vi "Actor Core.vi"(8 "Error In":errorcluster, 11 "BNT_SLTagMonitor in":refnum<class "BNT_SLTagMonitor.lvclass">) -> (0 "Error Out":errorcluster, 3 "Actor out":refnum<class "Actor.lvclass">)   [LabVIEW 2019, in "BNT_SLTagMonitor.lvlib" / "BNT_SLTagMonitor.lvclass"]
doc: "(<B>Filename</B>: Actor Framework.lvlib:Actor.lvclass:Actor Core.vi)\n\nReceives messages to the actor, reacts to them, and initiates any error handling that may shut the actor down.\n\nDescendant classes may override this VI to append parallel tasks for the actor to complete while it handles messages. Overrides use the Call Parent Method node."
uses:
  BNT_SLTagMonitor.lvclass
  CSPP_Core/Messages/CSPP_PVUpdate Msg/CSPP_PVUpdate Msg.lvclass
  CSPP_Core/Classes/CSPP_ProcessVariables/ProcessVariable/PV.lvclass
  CSPP_Core/Actors/CSPP_PVMonitor/CSPP_PVMonitor.lvclass
  CSPP_Core/Actors/CSPP_BaseActor/CSPP_BaseActor.lvclass
  C:/Users/Holger/Documents/LVP/CSPP/CSPP-Template/Packages/CSPP_Core/Actors/CSPP_PVMonitor/CSPP_PVMonitor.lvclass
  C:/Users/Holger/Documents/LVP/CSPP/CSPP-Template/Packages/CSPP_Core/Actors/CSPP_BaseActor/CSPP_BaseActor.lvclass
  C:/Program Files (x86)/National Instruments/LabVIEW 2019/vi.lib/ActorFramework/Actor/Actor.lvclass
  CSPP_Core/Actors/CSPP_BaseActor Messages/Open Actor Core FP Msg/Open Actor Core FP Msg.lvclass
  <vilib>/ActorFramework/Actor/Actor.lvclass
  <vilib>/Skyline/Tag/Wrapper/Wrapper_class/NI Skyline Tag.lvclass
  CSPP_Core/Libraries/Utilities/CSPP_Utilities.lvlib
  <vilib>/Skyline/Tag/Wrapper/Wrapper_class/Read Tag (Timestamp).vi
  <vilib>/Skyline/Tag/Wrapper/Wrapper_class/Read Tag (String).vi
  <vilib>/Skyline/Tag/Wrapper/Wrapper_class/Read Tag (I32).vi
  <vilib>/Skyline/Tag/Wrapper/Wrapper_class/Read Tag (DBL).vi
  <vilib>/Skyline/Tag/Wrapper/Wrapper_class/Read Tag (Boolean).vi
panel:
  out "Monitor Name":string
  out "Monitored PVs":string[](array[string])
  in  "Refresh Button":bool
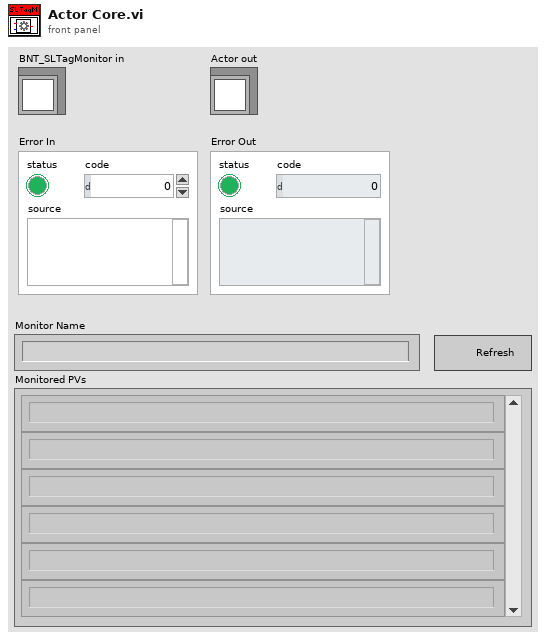
[diagram p1: front panel]
types:
  T1 = cluster{"Stop":refnum<user-event>, "PV Connections":refnum<user-event>}
  T2 = cluster{"Enqueuer":refnum<class "Message Enqueuer.lvclass">, "CSPP_PVUpdate Msg":refnum<class "CSPP_PVUpdate Msg.lvclass">}[]
  T3 = typedef "NI Skyline Tag.lvlib/DataType.ctl" = enum32{"Double", "I32", "String", "Boolean", "U64", "Timestamp"}
  T4 = cluster{"PV URL":string, "Observers":cluster{"Enqueuer":refnum<class "Message Enqueuer.lvclass">, "CSPP_PVUpdate Msg":refnum<class "CSPP_PVUpdate Msg.lvclass">}[]}[]
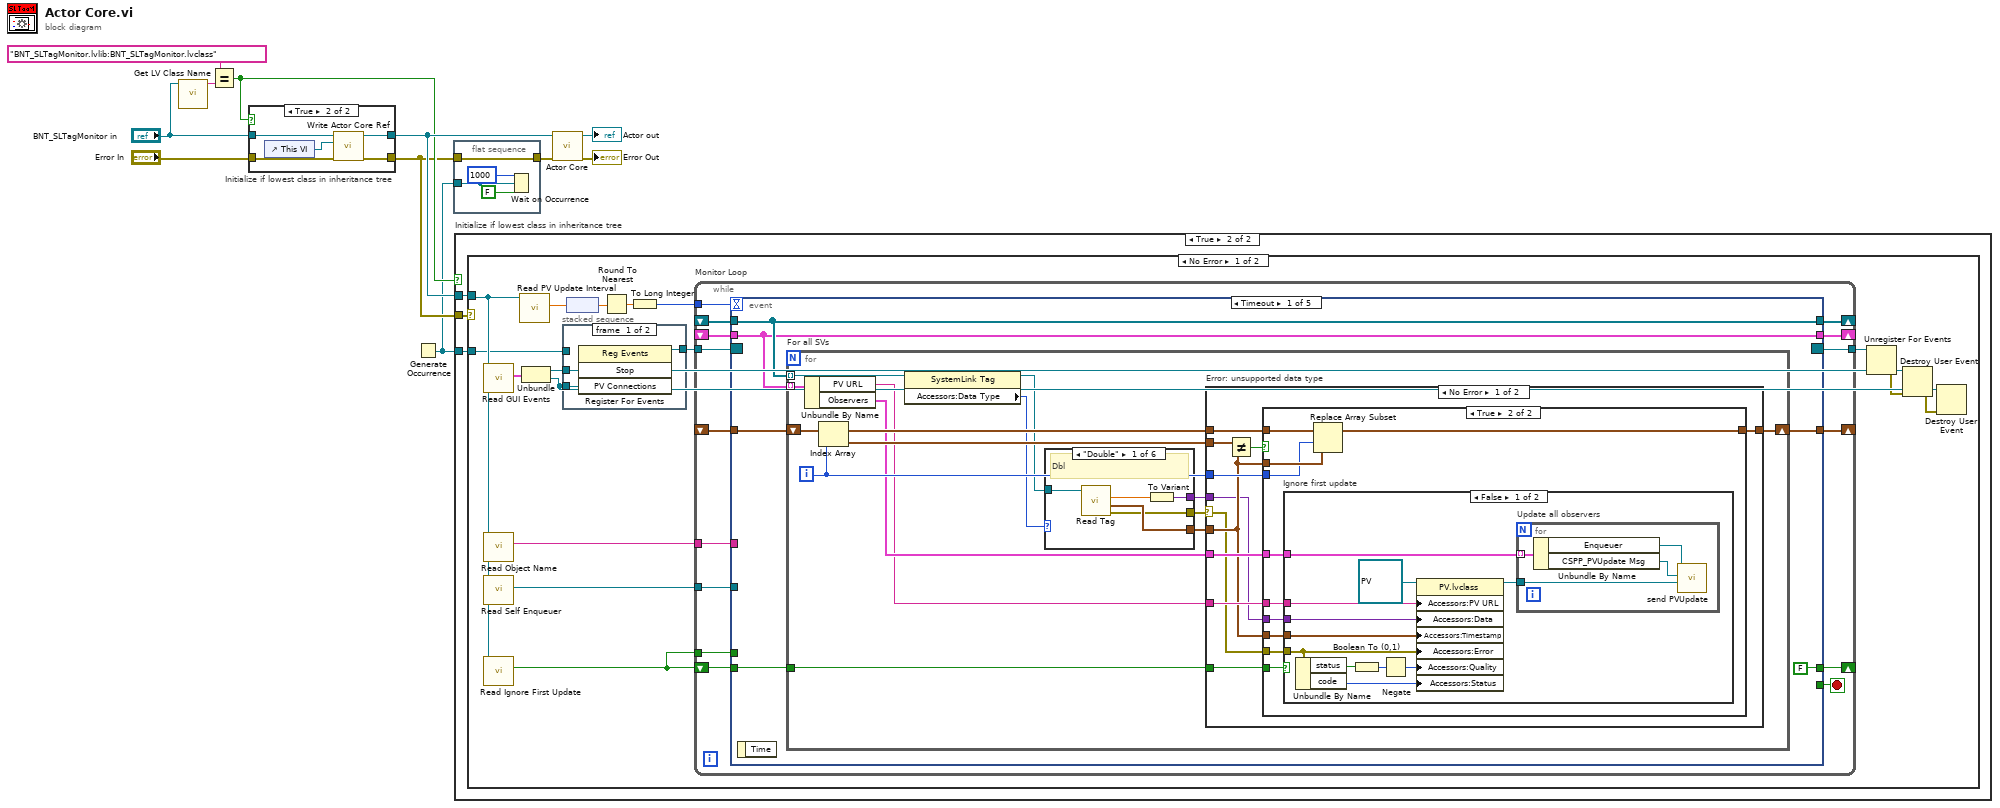
[diagram p0: block diagram]
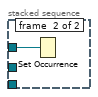
[diagram p4: hidden frame]
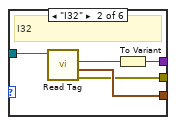
[diagram p8: hidden frame]
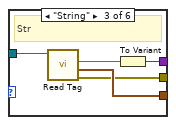
[diagram p9: hidden frame]
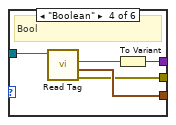
[diagram p10: hidden frame]
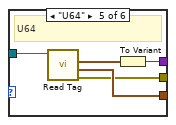
[diagram p11: hidden frame]
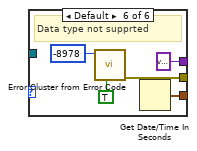
[diagram p12: hidden frame]
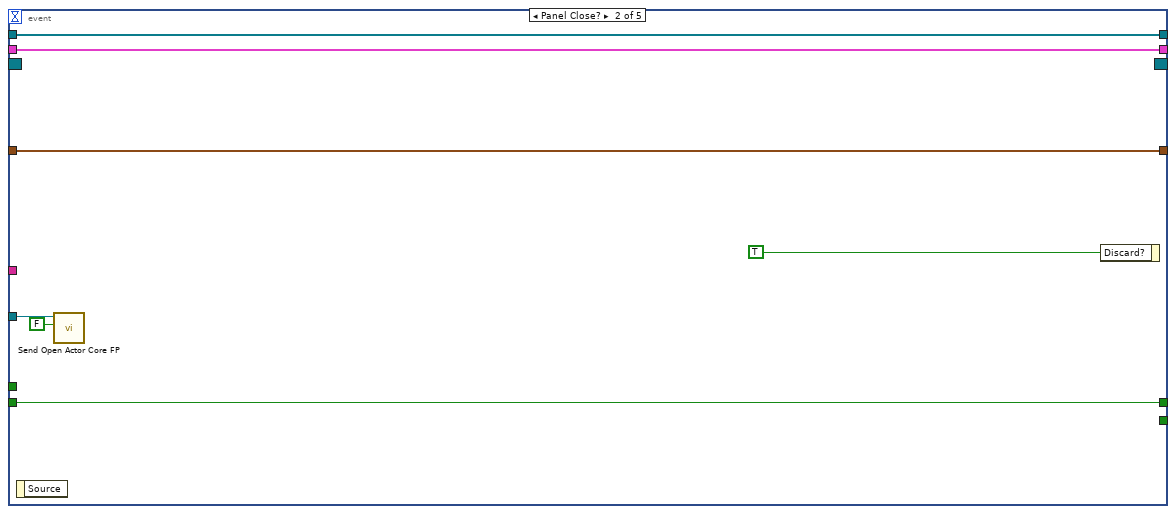
[diagram p13: hidden frame]
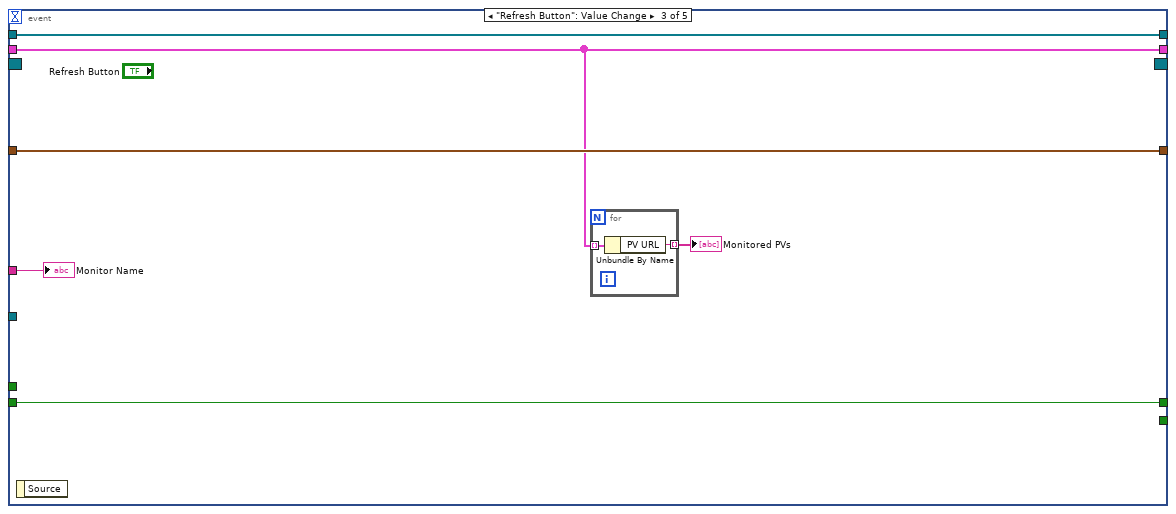
[diagram p14: hidden frame]
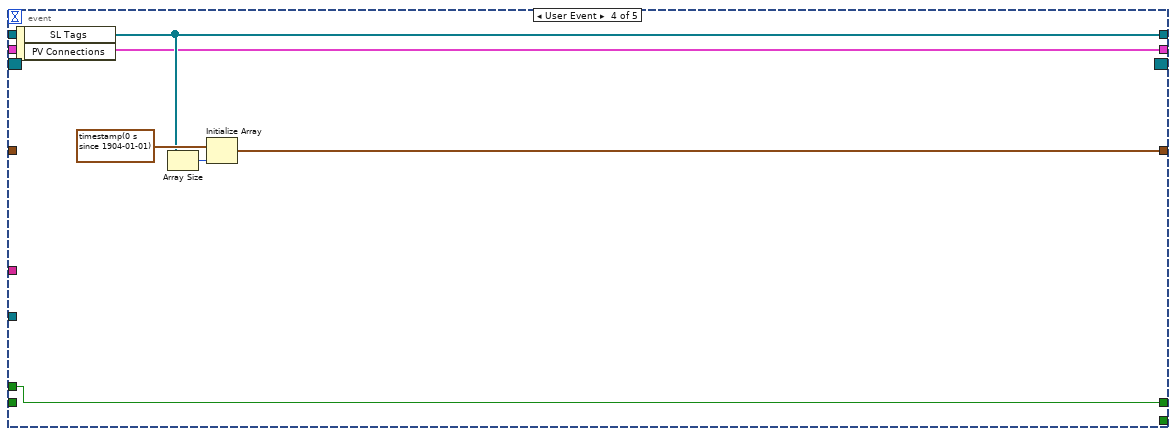
[diagram p15: hidden frame]
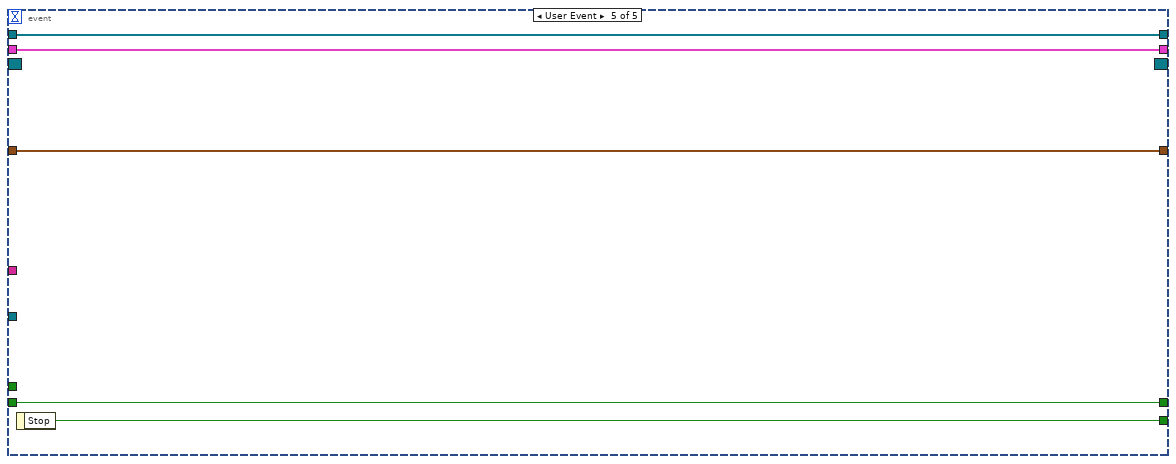
[diagram p16: hidden frame]
diagram:
  n1 = call <vilib>:"Get LV Class Name.vi"("object"="BNT_SLTagMonitor in") -> ("class name"=w9:string)  [unwired: 9 in, 1 out]
  n2 = Equal?(x="BNT_SLTagMonitor.lvlib:BNT_SLTagMonitor.lvclass" ("class name"), y=w9) -> (x = y?=w6:bool)
  n3 = case "Initialize if lowest class in inheritance tree" shown="True" w6 {
    tunnel: "BNT_SLTagMonitor in" -> [w13 w18]
    tunnel: [w12 w16] -> w5
    tunnel: "Error In" -> [w12 w14]
    tunnel: [w13 w17] -> w7
    frame False {
    }
    frame True {
      n4 = control-ref of="This VI"() -> (w15:refnum<vi>)
      n5 = call "Write Actor Core Ref.vi"("error in (no error)"=w14, "Actor Core Ref"=w15, "CSPP_BaseActor in"=w18) -> ("error out"=w16:errorcluster, "CSPP_BaseActor out"=w17:refnum<class "BNT_SLTagMonitor.lvclass">)  [unwired: 7 in]
    }
  }
  n6 = Generate Occurrence() -> (w3:refnum<k4>)
  n7 = flat-sequence {
    tunnel: w5 -> [w22]
    tunnel: [w22] -> w4
    tunnel: [w19] -> _
    tunnel: w3 -> [w19]
    frame #0 {
      n8 = Wait on Occurrence(1:FALSE ("ignore previous (T)"), 2:w19, 3:1000 ("ms timeout (-1)")) -> ()  [unwired: 1 out]
    }
  }
  n9 = case "Initialize if lowest class in inheritance tree" shown="True" w6 {
    tunnel: w5 -> [_ w25]
    tunnel: w7 -> [_ w24]
    tunnel: w3 -> [_ w23]
    frame False {
    }
    frame True {
      n10 = case shown="No Error" w25 {
        tunnel: w24 -> [w28 _]
        tunnel: w23 -> [w26 _]
        frame No Error {
          n11 = call "Read GUI Events.vi"("BNT_SLTagMonitor in"=w28) -> ("GUI Events"=w37:T1)  [unwired: 8 in, 2 out]
          n12 = call "Read Object Name.vi"("CSPP_BaseActor in"=w28) -> ("Object Name"=w27:string)  [unwired: 8 in, 2 out]
          n13 = call <vilib>:"Read Self Enqueuer.vi"("Actor"=w28) -> ("Self Enqueuer"=w29:refnum<class "Message Enqueuer.lvclass">)  [unwired: 10 in]
          n14 = call "Read Ignore First Update.vi"("CSPP_PVMonitor in"=w28) -> ("Ignore First Update"=w31:bool)  [unwired: 8 in, 2 out]
          n15 = call "Read PV Update Interval.vi"("CSPP_PVMonitor in"=w28) -> ("PV Update Interval"=w30:dbl[unit])  [unwired: 8 in, 2 out]
          n16 = Unbundle(w37) -> ("Stop"=w35:refnum<user-event>, "PV Connections"=w34:refnum<user-event>)
          n17 = stacked-sequence {
            tunnel: [w44 _] -> w38
            tunnel: w35 -> [w43 _]
            tunnel: w34 -> [w42 _]
            tunnel: w26 -> [_ w45]
            frame #0 {
              n18 = register-events(w43, w42) -> (reference out=w44:refnum<event-registration>)  [unwired: 2 in, 1 out]
            }
            frame #1 {
              n19 = Set Occurrence(w45) -> ()
            }
          }
          n20 = node(w30) -> (w40:dbl)
          n21 = Round To Nearest(number=w40) -> (nearest integer value=w41:dbl)
          n22 = To Long Integer(number=w41) -> (32bit integer=w39:i32)
          n23 = while "Monitor Loop" {
            tunnel: w38 -> [w60]
            tunnel: w39 -> [w59]
            tunnel: [w57] -> w36
            shift-right: [w55] -> _
            shift-left: _ -> [w56]
            shift-right: [w53] -> _
            shift-left: _ -> [w54]
            shift-right: [w52] -> _
            shift-left: _ -> [w51]
            shift-right: [w49] -> _
            shift-left: w31 -> [w50]
            tunnel: w31 -> [w48]
            tunnel: w29 -> [w47]
            tunnel: w27 -> [w46]
            stop <- w58 stop-if-true
            n24 = event shown="[0] Timeout" {
              selector: w60 -> [_ _ _ _ _]
              dyn-events: [_ _ _ _ _] -> w57
              timeout: w59 -> [_ _ _ _ _]
              tunnel: [_ _ _ _ w174] -> w58
              tunnel: w56 -> [w66 w152 w160 _ w173]
              tunnel: [w65 w152 w160 w166 w173] -> w55
              tunnel: w54 -> [w64 w154 w161 _ w172]
              tunnel: [w64 w154 w161 w167 w172] -> w53
              tunnel: [w63 w153 w158 w165 w171] -> w52
              tunnel: w51 -> [w63 w153 w158 _ w171]
              tunnel: w50 -> [w62 w151 w159 _ w170]
              tunnel: [FALSE w151 w159 w164 w170] -> w49
              tunnel: w48 -> [_ _ _ w164 _]
              tunnel: w47 -> [_ w149 _ _ _]
              tunnel: w46 -> [_ _ w156 _ _]
              event Timeout {
                n25 = event-data() -> ()  [unwired: 1 in, 1 out]
                n26 = for "For all SVs" {
                  shift-right: [w77] -> w65
                  shift-left: w66 -> [w79]
                  tunnel: w64 -> [w68] mode=indexing
                  tunnel: w63 -> [w76] mode=indexing
                  tunnel: w62 -> [w73]
                  i -> [w78]
                  n27 = Unbundle By Name(w76) -> ("PV URL"=w74:string, "Observers"=w75:T2)
                  n28 = Index Array(array=w79, index=w78) -> (element=w80:timestamp)
                  n29 = property class="SystemLink Tag"(reference=w68) -> (reference out=w69:refnum<class "NI Skyline Tag.lvclass">, "Accessors:Data Type"=w67:T3)  [unwired: 1 in, 1 out]
                  n30 = case shown="\"Double\"" w67 {
                    tunnel: w69 -> [w123 w128 w133 w138 w143 _]
                    tunnel: [w119 w124 w129 w134 w139 variant ("Variant")] -> w71
                    tunnel: [w121 w126 w131 w136 w141 w148] -> w72
                    tunnel: [w120 w125 w130 w135 w140 w144] -> w70
                    frame "Double" {
                      # "Dbl"
                      n31 = call-poly <vilib>:"Read Tag.vi"("tag in"=w123) -> ("error out"=w120:errorcluster, "time stamp"=w121:timestamp, "value"=w122:dbl)  [unwired: 6 in, 2 out]
                      n32 = To Variant(anything=w122) -> (Variant=w119:variant)
                    }
                    frame "I32" {
                      # "I32"
                      n33 = call-poly <vilib>:"Read Tag.vi"("tag in"=w128) -> ("error out"=w125:errorcluster, "time stamp"=w126:timestamp, "value"=w127:i32)  [unwired: 6 in, 2 out]
                      n34 = To Variant(anything=w127) -> (Variant=w124:variant)
                    }
                    frame "String" {
                      # "Str"
                      n35 = call-poly <vilib>:"Read Tag.vi"("tag in"=w133) -> ("error out"=w130:errorcluster, "time stamp"=w131:timestamp, "value"=w132:string)  [unwired: 6 in, 2 out]
                      n36 = To Variant(anything=w132) -> (Variant=w129:variant)
                    }
                    frame "Boolean" {
                      # "Bool"
                      n37 = call-poly <vilib>:"Read Tag.vi"("tag in"=w138) -> ("error out"=w135:errorcluster, "time stamp"=w136:timestamp, "value"=w137:bool)  [unwired: 6 in, 2 out]
                      n38 = To Variant(anything=w137) -> (Variant=w134:variant)
                    }
                    frame "U64" {
                      # "U64"
                      n39 = call-poly <vilib>:"Read Tag.vi"("tag in"=w143) -> ("error out"=w140:errorcluster, "time stamp"=w141:timestamp, "value"=w142:timestamp)  [unwired: 6 in, 2 out]
                      n40 = To Variant(anything=w142) -> (Variant=w139:variant)
                    }
                    frame Default {
                      # "Data type not supprted"
                      n41 = call "Error Cluster from Error Code.vi"("show call chain? (False)"=TRUE, "Error Code (0)"=-8978 ("error code (0)")) -> ("Error Out"=w144:errorcluster)  [unwired: 9 in]
                      n42 = Get Date/Time In Seconds() -> (seconds since 1Jan1904=w148:timestamp)
                    }
                  }
                  n43 = case "Error: unsupported data type" shown="No Error" w70 {
                    selector: w70 -> [w81 _]
                    tunnel: w80 -> [w91 _]
                    tunnel: w79 -> [w90 w118]
                    tunnel: w78 -> [w89 _]
                    tunnel: [w88 w118] -> w77
                    tunnel: w75 -> [w86 _]
                    tunnel: w74 -> [w85 _]
                    tunnel: w73 -> [w84 _]
                    tunnel: w72 -> [w83 _]
                    tunnel: w71 -> [w82 _]
                    frame No Error {
                      n44 = Not Equal?(x=w91, y=w83) -> (x != y?=w87:bool)
                      n45 = case shown="True" w87 {
                        tunnel: w83 -> [_ w102]
                        tunnel: w90 -> [w92 w101]
                        tunnel: w89 -> [_ w100]
                        tunnel: [w92 w99] -> w88
                        tunnel: w82 -> [_ w96]
                        tunnel: w83 -> [_ w95]
                        tunnel: w81 -> [_ w94]
                        tunnel: w86 -> [_ w98]
                        tunnel: w85 -> [_ w97]
                        tunnel: w84 -> [_ w93]
                        frame False {
                        }
                        frame True {
                          n46 = case "Ignore first update" shown="False" w93 {
                            tunnel: w98 -> [w113 _]
                            tunnel: w97 -> [w108 _]
                            tunnel: w96 -> [w107 _]
                            tunnel: w95 -> [w106 _]
                            tunnel: w94 -> [w105 _]
                            frame False {
                              n47 = Unbundle By Name(w105) -> ("status"=w109:bool, "code"=w112:i32)
                              n48 = Boolean To (0,1)(Boolean=w109) -> (0, 1=w110:i16)
                              n49 = Negate(x=w110) -> (-x=w111:i16)
                              n50 = property class="PV.lvclass"(reference=refnum<class "PV.lvclass"> refnum ("PV"), "Accessors:PV URL"=w108, "Accessors:Data"=w107, "Accessors:Timestamp"=w106, "Accessors:Error"=w105, "Accessors:Quality"=w111, "Accessors:Status"=w112) -> (reference out=w103:refnum<class "PV.lvclass">)  [unwired: 1 in, 1 out]
                              n51 = for "Update all observers" {
                                tunnel: w113 -> [w117] mode=indexing
                                tunnel: w103 -> [w114]
                                n52 = Unbundle By Name(w117) -> ("Enqueuer"=w116:refnum<class "Message Enqueuer.lvclass">, "CSPP_PVUpdate Msg"=w115:refnum<class "CSPP_PVUpdate Msg.lvclass">)
                                n53 = call "send PVUpdate.vi"("PV"=w114, "CSPP_PVUpdate Msg in"=w115, "Message Enqueuer in"=w116) -> ()  [unwired: 7 in, 2 out]
                              }
                            }
                            frame True {
                            }
                          }
                          n54 = Replace Array Subset(array=w101, new element=w102, index=w100) -> (w99:timestamp[])
                        }
                      }
                    }
                    frame Error {
                    }
                  }
                }
              }
              event Panel Close? {
                n55 = event-data() -> ()  [unwired: 1 in, 1 out]
                n56 = call "Send Open Actor Core FP.vi"("Open FP (F)"=FALSE, "Message Enqueuer"=w149) -> ()  [unwired: 8 in, 2 out]
                n57 = event-data("Discard?"=TRUE) -> ()  [unwired: 1 in, 1 out]
              }
              event "Refresh Button": Value Change {
                n58 = event-data() -> ()  [unwired: 1 in, 1 out]
                n59 = for {
                  tunnel: w158 -> [w163] mode=indexing
                  tunnel: [w162] -> w157 mode=indexing
                  n60 = Unbundle By Name(w163) -> ("PV URL"=w162:string)
                }
                "Monitored PVs" <- w157
                "Monitor Name" <- w156
              }
              event User Event {
                n61 = event-data() -> ("SL Tags"=w167:refnum<class "NI Skyline Tag.lvclass">[], "PV Connections"=w165:T4)  [unwired: 1 in]
                n62 = Array Size(array=w167) -> (size(s)=w169:i32)
                n63 = Initialize Array(timestamp(0 s since 1904-01-01) ("timestamp"), w169) -> (w166:timestamp[])
              }
              event User Event {
                n64 = event-data() -> ("Stop"=w174:bool)  [unwired: 1 in]
              }
            }
          }
          n65 = Unregister For Events(event registration refnum=w36) -> (error out=w33:errorcluster)  [unwired: 1 in]
          n66 = Destroy User Event(user event=w35, error in=w33) -> (error out=w32:errorcluster)
          n67 = Destroy User Event(user event=w34, error in=w32) -> ()  [unwired: 1 out]
        }
        frame Error {
        }
      }
    }
  }
  n68 = call-parent "Actor Core.vi"("error in"=w4, "CSPP_BaseActor in"=w7) -> ("error out"=→"Error Out":errorcluster, "Actor out"=→"Actor out":refnum<class "Actor.lvclass">)  [unwired: 8 in]
